vi "sort_error.vi"(0 "check_error":errorcluster, 11 "error constant":errorcluster) -> (4 "output cluster":T2, 15 "error out":errorcluster)   [LabVIEW 2023]
doc: "Used to sort the error and extract the necessary details"
uses:
  Controls/errors_type.ctl
  Controls/error_cluster.ctl
  <vilib>/regexp/Match Regular Expression.xnode
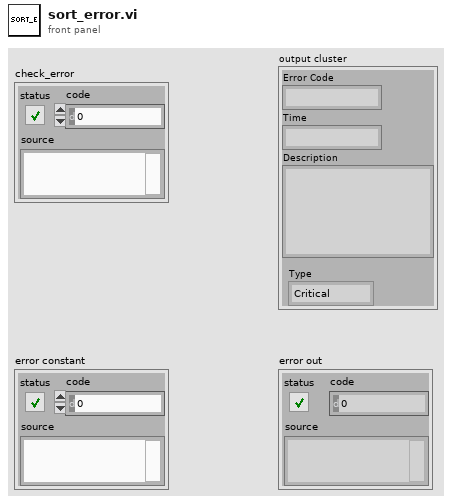
[diagram p1: front panel]
types:
  T1 = typedef "errors_type.ctl" = enum16{"Critical", "No error", "Warning", "Passive", "Unknown"}
  T2 = cluster{"Error Code":string, "Time":string, "Description":string, "Type":T1}
  T3 = typedef "error_cluster.ctl" = cluster{"Error Code":string, "Time":string, "Description":string, "Type":T1}
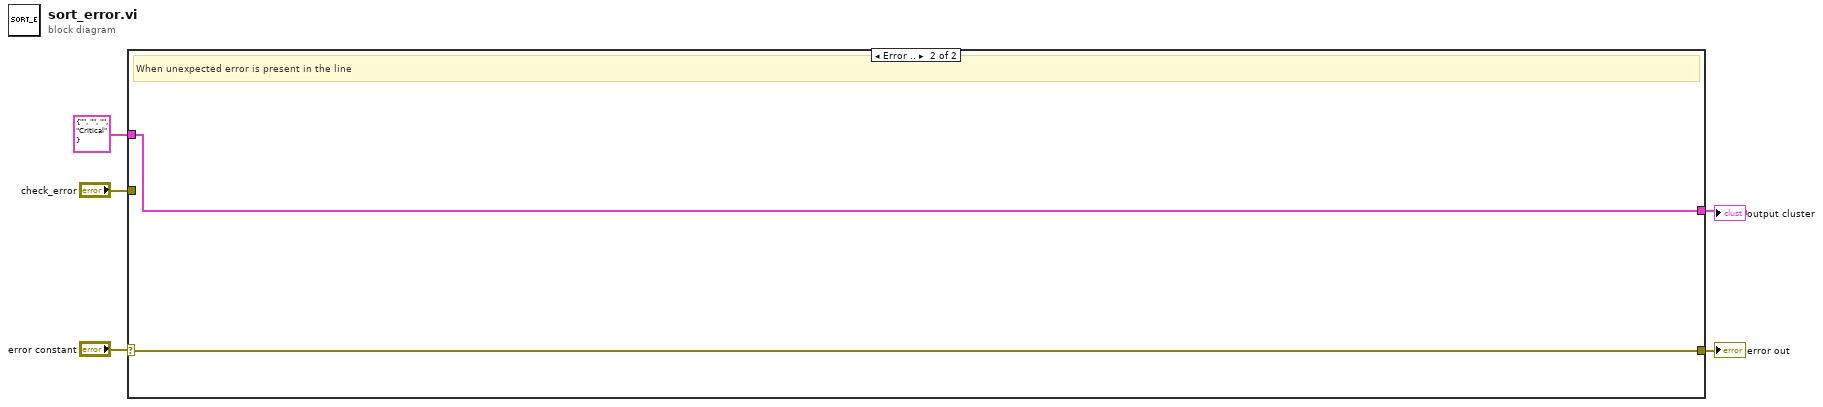
[diagram p0: block diagram]
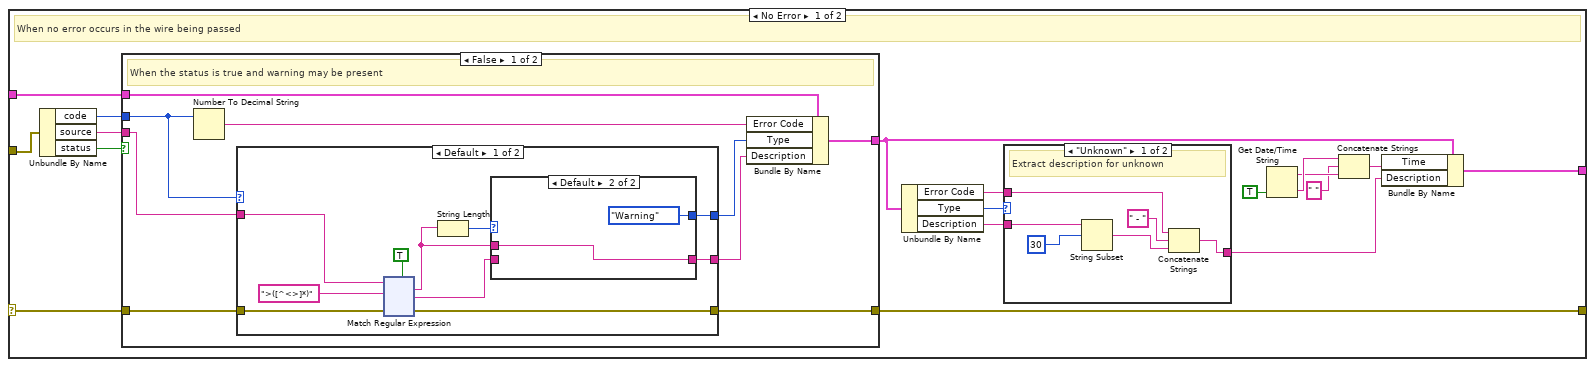
[diagram p2: hidden frame]
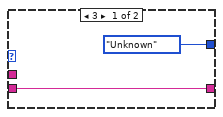
[diagram p3: hidden frame]
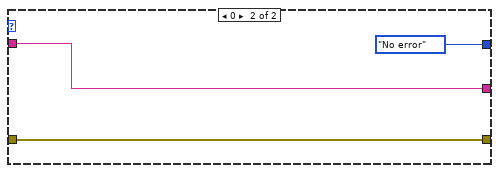
[diagram p4: hidden frame]
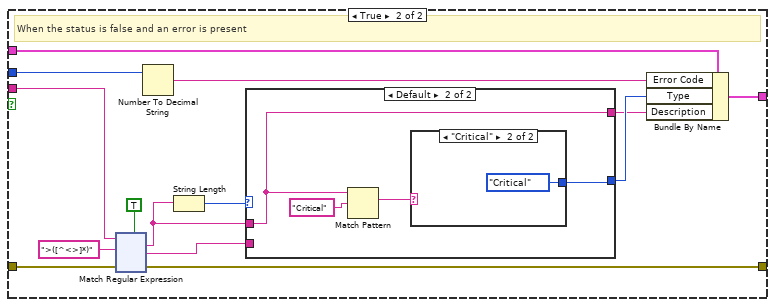
[diagram p5: hidden frame]
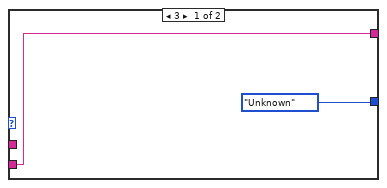
[diagram p6: hidden frame]
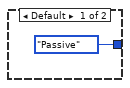
[diagram p7: hidden frame]
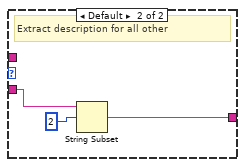
[diagram p8: hidden frame]
diagram:
  n1 = case shown="Error .." "error constant" {
    selector: "error constant" -> [w19 w316]
    tunnel: [w18 w316] -> w4
    tunnel: T3 {"Error Code"="", "Time"="", "Description"="", "Type"=enum."Critical"} -> [w23 w315]
    tunnel: "check_error" -> [w9 _]
    tunnel: [w6 w315] -> w1
    frame No Error {
      # "When no error occurs in the wire being passed"
      n2 = Unbundle By Name(w9) -> ("code"=w22:i32, "source"=w21:string, "status"=w20:bool)
      n3 = case shown="False" w20 {
        tunnel: w23 -> [w32 w171]
        tunnel: [w30 w172] -> w10
        tunnel: w22 -> [w29 w170]
        tunnel: w21 -> [w27 w169]
        tunnel: w19 -> [w25 w168]
        tunnel: [w24 w167] -> w18
        frame False {
          # "When the status is true and warning may be present"
          n4 = Number To Decimal String(number=w29) -> (decimal integer string=w31:string)  [unwired: 1 in]
          n5 = case shown="Default" w29 {
            tunnel: w27 -> [w38 w165]
            tunnel: [w39 errors_type."No error" ("Type")] -> w28
            tunnel: [w36 w165] -> w26
            tunnel: w25 -> [w34 w164]
            tunnel: [w33 w164] -> w24
            frame Default {
              n6 = xnode "Match Regular Expression"("input string"=w38, "regular expression"=">([^<>]*)", "error in"=w34, "multiline? (F)"=TRUE) -> ("whole match"=w37:string, "after match"=w35:string, "error out"=w33:errorcluster)  [unwired: 2 in, 2 out]
              n7 = String Length(string=w37) -> (length=w40:i32)
              n8 = case shown="Default" w40 {
                tunnel: w37 -> [_ w162]
                tunnel: [errors_type."Unknown" ("Type") errors_type."Warning" ("Type")] -> w39
                tunnel: [w160 w162] -> w36
                tunnel: w35 -> [w160 _]
                frame 3 {
                }
                frame Default {
                }
              }
            }
            frame 0 {
            }
          }
          n9 = Bundle By Name(cluster=w32, "Error Code"=w31, "Type"=w28, "Description"=w26) -> (w30:T3)
        }
        frame True {
          # "When the status is false and an error is present"
          n10 = xnode "Match Regular Expression"("input string"=w169, "regular expression"=">([^<>]*)", "error in"=w168, "multiline? (F)"=TRUE) -> ("whole match"=w177:string, "after match"=w175:string, "error out"=w167:errorcluster)  [unwired: 2 in, 2 out]
          n11 = Number To Decimal String(number=w170) -> (decimal integer string=w178:string)  [unwired: 1 in]
          n12 = String Length(string=w177) -> (length=w180:i32)
          n13 = case shown="Default" w180 {
            tunnel: [errors_type."Unknown" w301] -> w179
            tunnel: w177 -> [_ w300]
            tunnel: [w298 w300] -> w176
            tunnel: w175 -> [w298 _]
            frame 3 {
            }
            frame Default {
              n14 = Match Pattern(string=w300, regular expression="Critical") -> (match substring=w302:string)  [unwired: 1 in, 3 out]
              n15 = case shown="\"Critical\"" w302 {
                tunnel: [errors_type."Passive" errors_type."Critical"] -> w301
                frame Default {
                }
                frame "Critical" {
                }
              }
            }
          }
          n16 = Bundle By Name(cluster=w171, "Error Code"=w178, "Type"=w179, "Description"=w176) -> (w172:T3)
        }
      }
      n17 = Unbundle By Name(w10) -> ("Error Code"=w17:string, "Type"=w15:T1, "Description"=w16:string)
      n18 = case shown="\"Unknown\"" w15 {
        tunnel: [w311 w313] -> w14
        tunnel: w16 -> [w309 w312]
        tunnel: w17 -> [w308 _]
        frame "Unknown" {
          # "Extract description for unknown"
          n19 = String Subset(string=w309, offset (0)=30) -> (substring=w307:string)  [unwired: 1 in]
          n20 = Concatenate Strings(w308, " - " ("string"), w307) -> (w311:string)
        }
        frame Default {
          # "Extract description for all other"
          n21 = String Subset(string=w312, offset (0)=2) -> (substring=w313:string)  [unwired: 1 in]
        }
      }
      n22 = Get Date/Time String(want seconds? (F)=TRUE) -> (date string=w8:string, time string=w12:string)  [unwired: 2 in]
      n23 = Concatenate Strings(w12, " " ("string"), w8) -> (w13:string)
      n24 = Bundle By Name(cluster=w10, "Time"=w13, "Description"=w14) -> (w6:T3)
    }
    frame Error {
      # "When unexpected error is present in the line"
    }
  }
  "error out" <- w4
  "output cluster" <- w1
